vi "CB Range Check.vi"(9 "Actual Value":dbl, 10 "Acceptable% Error":dbl, 11 "Expected Value":dbl) -> (0 "Result (Boolean)":bool, 1 "Result (String)":string, 3 "Result (Color)":u32)   [LabVIEW 2022 SP3]
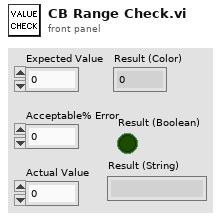
[diagram p1: front panel]
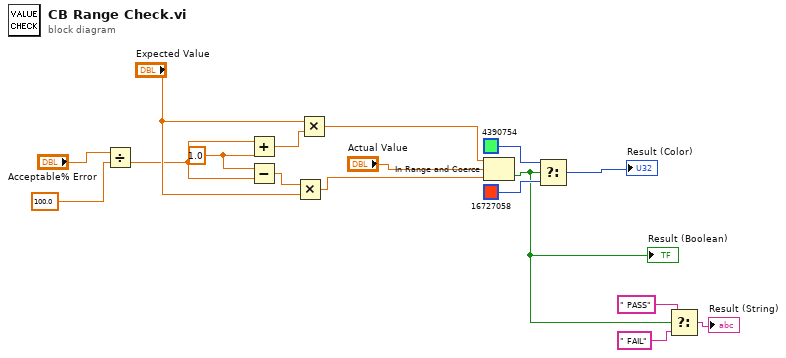
[diagram p0: block diagram]
diagram:
  w12 = 1.0
  n1 = Divide(x="Acceptable% Error", y=100.0) -> (x/y=w3:dbl)
  n2 = Add(x=w3, y=w12) -> (x+y=w16:dbl)
  n3 = Subtract(x=w12, y=w3) -> (x-y=w13:dbl)
  n4 = Multiply(x=w13, y="Expected Value") -> (x*y=w14:dbl)
  n5 = Multiply(x="Expected Value", y=w16) -> (x*y=w15:dbl)
  n6 = In Range and Coerce(upper limit=w15, x="Actual Value", lower limit=w14) -> (In Range?=w5:bool)  [unwired: 1 out]
  "Result (Boolean)" <- w5
  n7 = Select(t=u32 4390754, s=w5, f=u32 16727058) -> (s? t:f=→"Result (Color)":u32)
  n8 = Select(t=" PASS", s=w5, f=" FAIL") -> (s? t:f=→"Result (String)":string)
